vi "Less Than.vi"(1 "comparable b":string, 2 "comparable a":string, 3 "Less Functor":refnum<class "Numeric Strings Less Functor.lvclass">) -> (0 "less?":bool)   [LabVIEW 2023, in "Numeric Strings Less Functor.lvclass"]
doc: "Returns whether <b>comparable a</b> is less than <b>comparable b</b> by using Scan From String for a leading numeric value and sorting by that value. Two strings with the same numerical value are compared as equal, regardless of the rest of the string. Strings with leading numbers are considered less than strings without leading numbers."
uses:
  Numeric Strings Less Functor.lvclass
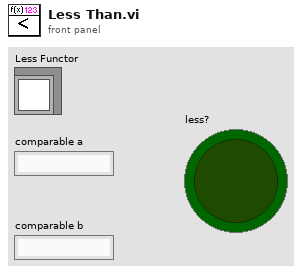
[diagram p1: front panel]
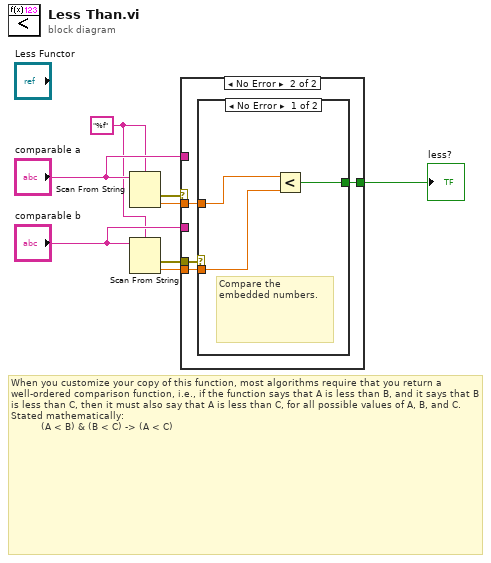
[diagram p0: block diagram]
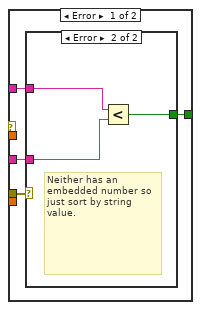
[diagram p2: hidden frame]
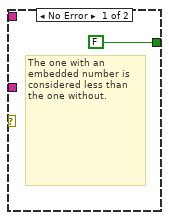
[diagram p3: hidden frame]
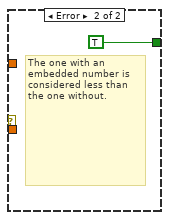
[diagram p4: hidden frame]
diagram:
  w1 = "%f" ("format string")
  # "When you customize your copy of this function, most algorithms require that you return a well-ordered comparison function, i.e., if the function says that A is less than B, and it says that B is less than C, then it must also say that A is less than C, for all possible values of A, B, and C. Stated mathematically:\n          (A < B) & (B < C) -> (A < C)"
  n1 = Scan From String(format string=w1, input string="comparable a") -> (error out=w8:errorcluster, output 1=w2:dbl)  [unwired: 3 in, 2 out]
  n2 = Scan From String(format string=w1, input string="comparable b") -> (error out=w7:errorcluster, output 1=w3:dbl)  [unwired: 3 in, 2 out]
  n3 = case shown="No Error" w8 {
    tunnel: w7 -> [w12 w20]
    tunnel: [w11 w19] -> w6
    tunnel: "comparable a" -> [w10 _]
    tunnel: "comparable b" -> [w9 _]
    tunnel: w3 -> [_ w18]
    tunnel: w2 -> [_ w17]
    frame Error {
      n4 = case shown="Error" w12 {
        tunnel: [FALSE w16] -> w11
        tunnel: w10 -> [_ w15]
        tunnel: w9 -> [_ w14]
        frame No Error {
          # "The one with an embedded number is considered less than the one without."
        }
        frame Error {
          # "Neither has an embedded number so just sort by string value."
          n5 = Less?(x=w15, y=w14) -> (x < y?=w16:bool)
        }
      }
    }
    frame No Error {
      n6 = case shown="No Error" w20 {
        tunnel: [w23 TRUE] -> w19
        tunnel: w18 -> [w22 _]
        tunnel: w17 -> [w21 _]
        frame No Error {
          # "Compare the embedded numbers."
          n7 = Less?(x=w21, y=w22) -> (x < y?=w23:bool)
        }
        frame Error {
          # "The one with an embedded number is considered less than the one without."
        }
      }
    }
  }
  "less?" <- w6
